vi "autoupdate.vi"   [LabVIEW 2016, in "数据传输系统.lvlib"]
uses:
  <vilib>/Utility/error.llb/whitespace.ctl
  update/update.lvlib
types:
  T1 = typedef "whitespace.ctl" = u16
  T2 = cluster{"主机":string, "用户":string, "密码":string, "远程路径":string, "下载文件名":string, "软件版本":string}
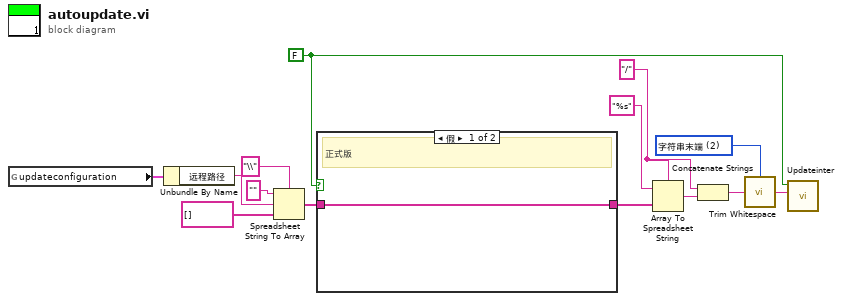
[diagram p0: block diagram]
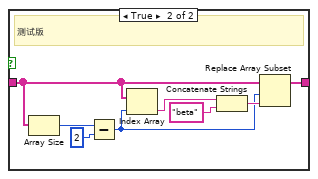
[diagram p2: hidden frame]
diagram:
  w11 = T1 2 items=["两端", "字符串首端", "字符串末端"] ("location (both)")
  w9 = "/" ("分隔符(Tab)")
  w2 = FALSE ("测试版？")
  n1 = global read "断电保存全局.vi" "updateconfiguration"() -> (w3:T2)
  n2 = Unbundle By Name(w3) -> ("远程路径"=w4:string)
  n3 = Spreadsheet String To Array(delimiter (Tab)="\\" ("分隔符(Tab)"), format string="" ("格式字符串"), spreadsheet string=w4, array type (2D Dbl)=string[] []) -> (array=w6:string[])
  n4 = case shown="假" w2 {
    tunnel: w6 -> [w15 w17]
    tunnel: [w15 w16] -> w5
    frame False {
      # "正式版"
    }
    frame True {
      # "测试版"
      n5 = Array Size(array=w17) -> (size(s)=w18:i32)
      n6 = Subtract(x=w18, y=2) -> (x-y=w20:i32)
      n7 = Index Array(array=w17, index=w20) -> (element=w21:string)
      n8 = Concatenate Strings(w21, "beta" ("字符串")) -> (w23:string)
      n9 = Replace Array Subset(array=w17, new element=w23, index=w20) -> (w16:string[])
    }
  }
  n10 = Array To Spreadsheet String(delimiter (Tab)=w9, array=w5, 3:"%s" ("格式字符串")) -> (spreadsheet string=w8:string)
  n11 = Concatenate Strings(w9, w8) -> (w7:string)
  n12 = call <vilib>:"Trim Whitespace.vi"("string"=w7, "location (both)"=w11) -> ("trimmed string"=w1:string)
  n13 = call "Updateinter.vi"("更新包远端地址"=w1, "测试版？"=w2) -> ()  [unwired: 10 in]
